vi "Query Error Count.vi"(8 "error in (no error)":errorcluster, 11 "VISA resource name":refnum<visa-resource-name>) -> (0 "error out":errorcluster, 2 "Error Count":i32, 3 "VISA resource name out":refnum<visa-resource-name>)   [LabVIEW 2020, in "Keithley 2600 Series.lvlib"]
doc: "Returns the error message count of the error queue."
uses:
  <instrlib>/Keithley 2600 Series/Keithley 2600 Series.lvlib
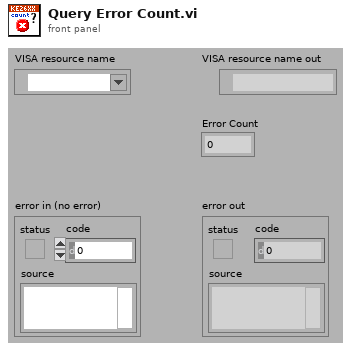
[diagram p1: front panel]
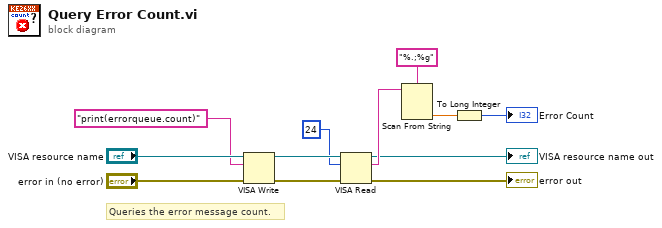
[diagram p0: block diagram]
diagram:
  # "Queries the error message count."
  n1 = VISA Write(VISA resource name="VISA resource name", write buffer="print(errorqueue.count)", error in (no error)="error in (no error)") -> (VISA resource name out=w10:refnum<visa-resource-name>, error out=w9:errorcluster)  [unwired: 1 out]
  n2 = VISA Read(VISA resource name=w10, byte count=u32 24, error in (no error)=w9) -> (VISA resource name out=→"VISA resource name out":refnum<visa-resource-name>, read buffer=w6:string, error out=→"error out":errorcluster)  [unwired: 1 out]
  n3 = Scan From String(format string="%.;%g", input string=w6) -> (output 1=w3:dbl)  [unwired: 3 in, 3 out]
  n4 = To Long Integer(number=w3) -> (32bit integer=→"Error Count":i32)
